vi "SetParam.vi"(8 "error in (no error)":errorcluster caption="entrée d'erreur (pas d'erreur)", 10 "normalize":T1={"norm"="l2", "axis"=1, "copy"=TRUE, "Returns"="X"}, 11 "normalize.lvclass":refnum<class "normalize.lvclass">) -> (0 "error out":errorcluster caption="sortie d'erreur", 3 "normalize.lvclass":refnum<class "normalize.lvclass">)   [LabVIEW 2020, in "normalize.lvclass"]
doc: "Set Parameters"
uses:
  normalize.lvclass
  normalize.lvclass/normalize.ctl
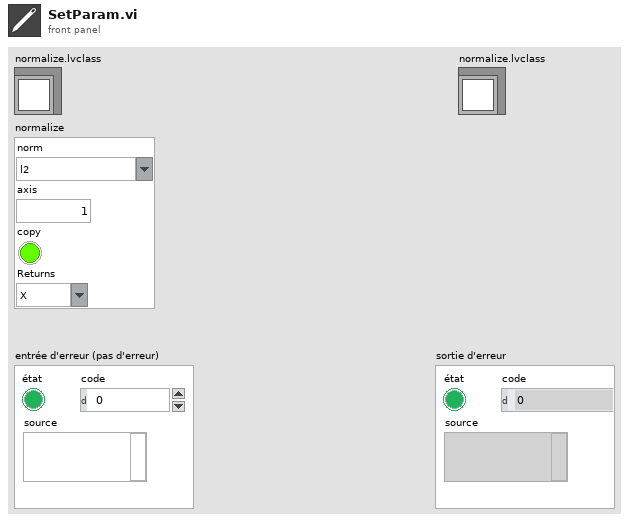
[diagram p1: front panel]
types:
  T1 = cluster{"norm":string, "axis":i32, "copy":bool, "Returns":string}
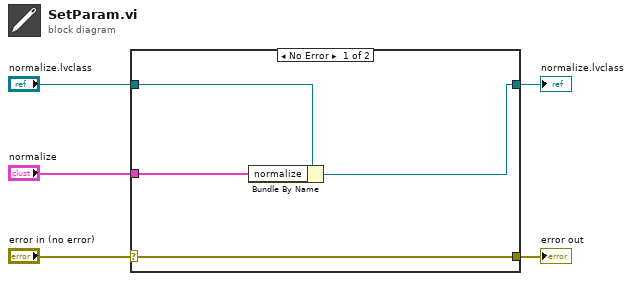
[diagram p0: block diagram]
diagram:
  n1 = case shown="No Error" "error in (no error)" {
    selector: "error in (no error)" -> [w9 w10]
    tunnel: [w9 w10] -> w4
    tunnel: [w7 w11] -> w2
    tunnel: "normalize.lvclass" -> [w8 w11]
    tunnel: "normalize" -> [w6 _]
    frame No Error {
      n2 = Bundle By Name(cluster=w8, "normalize"=w6) -> (w7:refnum<class "normalize.lvclass">)
    }
    frame Error {
    }
  }
  "error out" <- w4
  "normalize.lvclass" <- w2
